vi "Strip Units__ogtk.vi"(8 "error in (no error)":errorcluster, 10 "Number or 1D array with units":variant) -> (0 "error out":errorcluster, 2 "Pure Number(s) (base units)":variant)   [LabVIEW 2023, in "openg_variant.lvlib"]
doc: "Converts a number with or without units to pure number."
uses:
  openg_variant.lvlib
  error/error.llb/openg_error.lvlib
panel:
  # "[OpenG VI Tags] ***Do Not Remove***"
  # "Please visit http://www.OpenG.org to learn about the\nOpen Source LabVIEW software movement.\n\nNOTICE -- YOU MUST LEAVE THIS NOTICE IN PLACE.  PER THE TERMS OF THE LICENSE BELOW, YOU MAY SUBLICENSE THIS SOFTWARE \nIN ANY WAY THAT DOES NOT CONFLICT WITH THIS LICENSE.\n\n### BSD License (http://www.opensource.org/licenses/bsd-license.php) Begin ###\n \nCopyright (c) 2003, Jean-Pierre Drolet <drolet_jp@hotmail.com>\nCopyright (c) 2003-2006, Jim Kring <jim@jimkring.com>\n\nAll rights reserved.\n\nRedistribution and use in source and binary forms, with or without modification, are permitted provided that the following conditions are met:\n\n    * Redistributions of source code must retain the above copyright notice, this list of conditions and the following disclaimer.\n    * Redistributions in binary form must reproduce the above copyright notice, this list of conditions and the following disclaimer in the \n       documentation and/or other materials provided with the distribution.\n    * Neither the name of SciWare, James Kring, Inc., nor the names of its contributors may be used to endorse or promote products derived \n       from this software without specific prior written permission.\n\nTHIS SOFTWARE IS PROVIDED BY THE COPYRIGHT HOLDERS AND CONTRIBUTORS \"AS IS\" AND ANY EXPRESS OR IMPLIED WARRANTIES, \nINCLUDING, BUT NOT LIMITED TO, THE IMPLIED WARRANTIES OF MERCHANTABILITY AND FITNESS FOR A PARTICULAR PURPOSE ARE \nDISCLAIMED. IN NO EVENT SHALL THE COPYRIGHT OWNER OR CONTRIBUTORS BE LIABLE FOR ANY DIRECT, INDIRECT, INCIDENTAL,\n SPECIAL, EXEMPLARY, OR CONSEQUENTIAL DAMAGES (INCLUDING, BUT NOT LIMITED TO, PROCUREMENT OF SUBSTITUTE GOODS OR \nSERVICES; LOSS OF USE, DATA, OR PROFITS; OR BUSINESS INTERRUPTION) HOWEVER CAUSED AND ON ANY THEORY OF LIABILITY, \nWHETHER IN CONTRACT, STRICT LIABILITY, OR TORT (INCLUDING NEGLIGENCE OR OTHERWISE) ARISING IN ANY WAY OUT OF THE USE \nOF THIS SOFTWARE, EVEN IF ADVISED OF THE POSSIBILITY OF SUCH DAMAGE.\n\n### BSD License End ###"
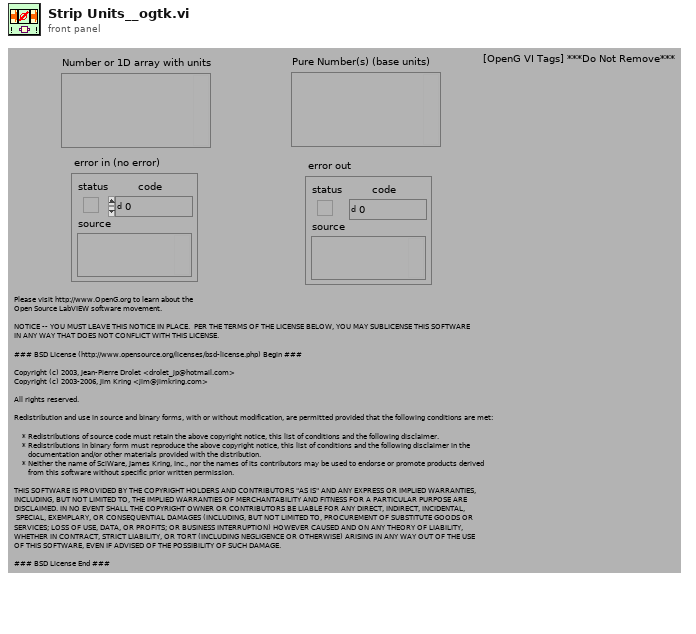
[diagram p1: front panel]
types:
  T1 = typedef "openg_variant.lvlib/Type Descriptor Header__ogtk.ctl" = cluster{"length":u16, "private":u8, "type":T2, "# elements":u16}
  T2 = typedef "openg_variant.lvlib/Type Descriptor Enumeration__ogtk.ctl" = enum8{"<Null>", "I8", "I16", "I32", "I64", "U8", "U16", "U32", "U64", "SGL", "DBL", "EXT", "CSG", "CDB", "CXT", "0x0F", "0x10", "0x11", "0x12", "0x13", "0x14", "Enum U8", "Enum U16", "Enum U32", "Enum U64", "SGL PQ", "DBL PQ", "EXT PQ", "CSG PQ", "CDB PQ", "CXT PQ", "0x1F", "0x20", "Boolean", "0x22", "0x23", "0x24", "0x25", "0x26", "0x27", "0x28", "0x29", "0x2A", "0x2B", "0x2C", "0x2D", "0x2E", "0x2F", "String", "0x31", "Path", "Pict", "0x34", "0x35", "0x36", "DAQ", "0x38", "0x39", "0x3A", "0x3B", "0x3C", "0x3D", "0x3E", "0x3F", "Array", "0x41", "0x42", "0x43", "0x44", "0x45", "0x46", "0x47", "0x48", "0x49", "0x4A", "0x4B", "0x4C", "0x4D", "0x4E", "0x4F", "Cluster", "0x51", "0x52", "Variant", "Waveform", "0x55", "0x56", "0x57", "0x58", "0x59", "0x5A", "0x5B", "0x5C", "0x5D", "0x5E", "Fixed Point", "0x60", "0x61", "0x62", "0x63", "0x64", "0x65", "0x66", "0x67", "0x68", "0x69", "0x6A", "0x6B", "0x6C", "0x6D", "0x6E", "0x6F", "Refnum", "0x71", "0x72", "Set Collection", "Map Collection"}
  T3 = typedef "openg_variant.lvlib/Type Descriptor__ogtk.ctl" = i16[]
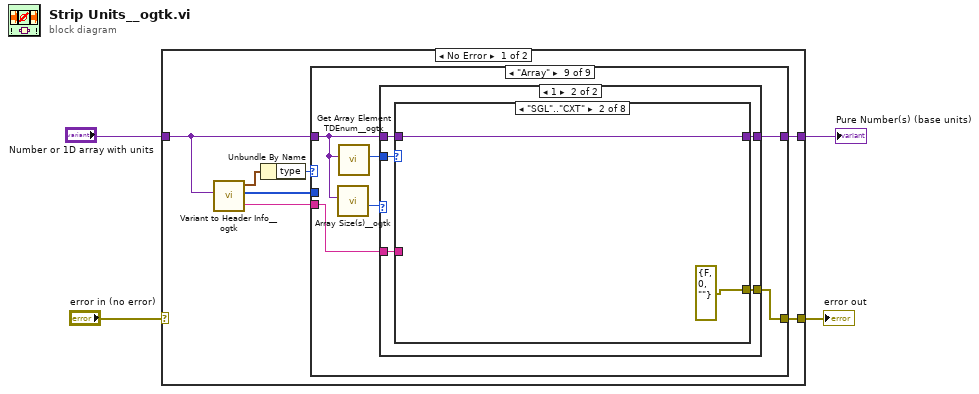
[diagram p0: block diagram]
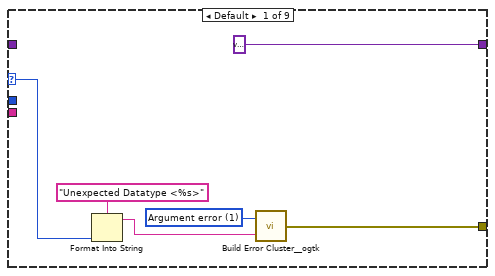
[diagram p2: hidden frame]
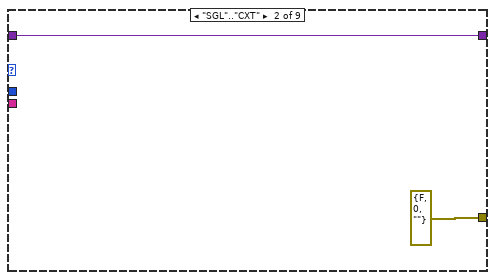
[diagram p3: hidden frame]
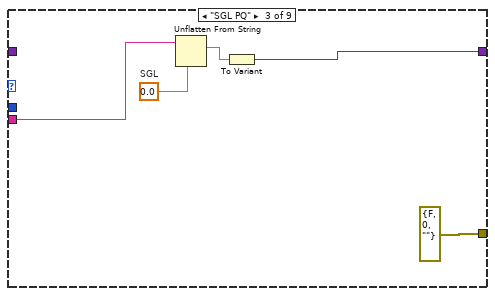
[diagram p4: hidden frame]
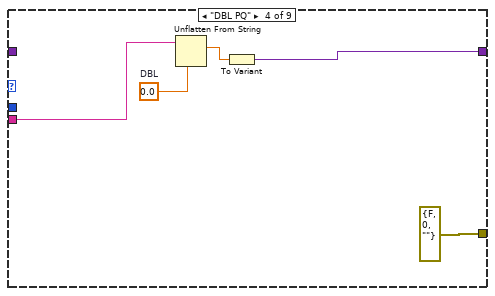
[diagram p5: hidden frame]
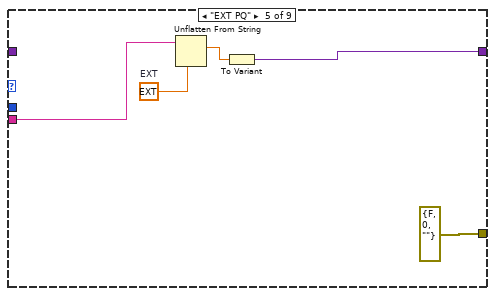
[diagram p6: hidden frame]
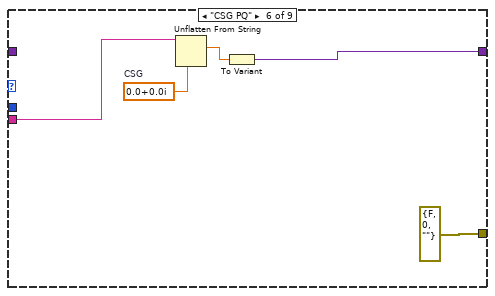
[diagram p7: hidden frame]
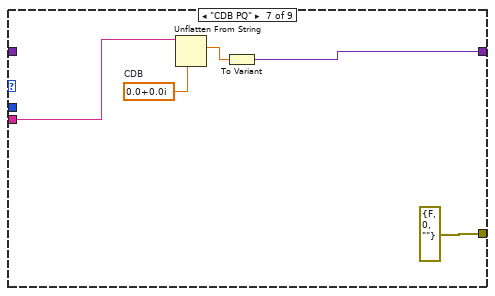
[diagram p8: hidden frame]
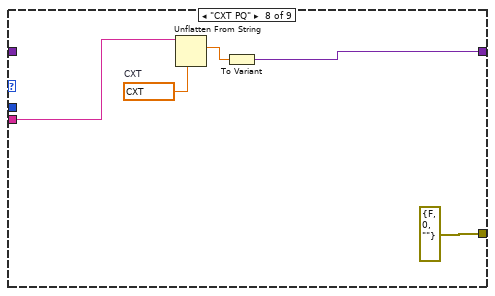
[diagram p9: hidden frame]
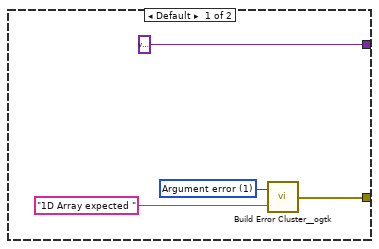
[diagram p10: hidden frame]
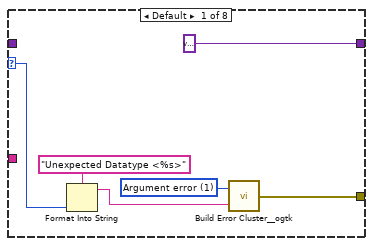
[diagram p11: hidden frame]
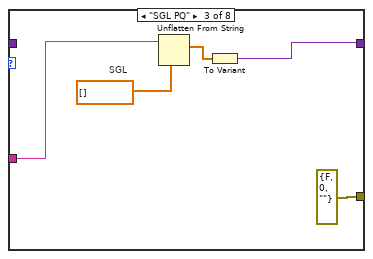
[diagram p12: hidden frame]
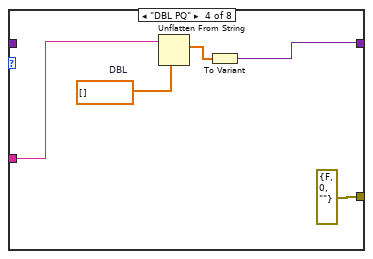
[diagram p13: hidden frame]
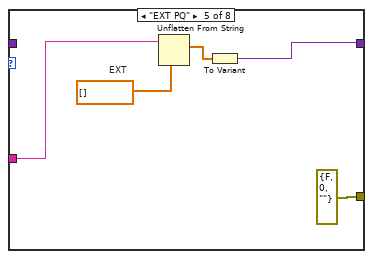
[diagram p14: hidden frame]
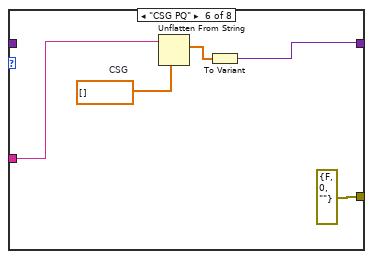
[diagram p15: hidden frame]
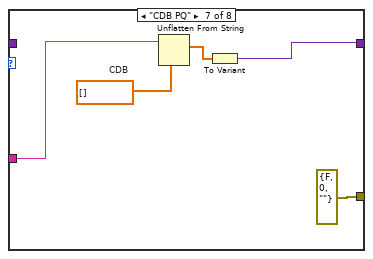
[diagram p16: hidden frame]
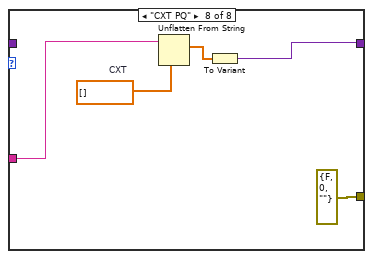
[diagram p17: hidden frame]
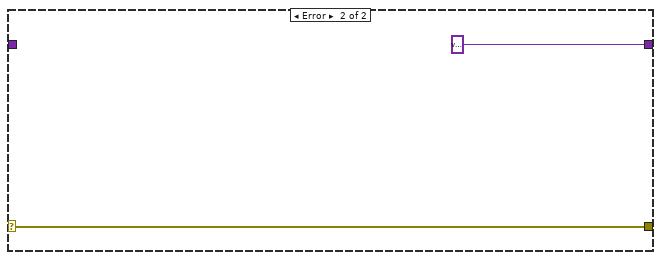
[diagram p18: hidden frame]
diagram:
  n1 = case shown="No Error" "error in (no error)" {
    selector: "error in (no error)" -> [_ w104]
    tunnel: [w11 w104] -> w4
    tunnel: "Number or 1D array with units" -> [w5 _]
    tunnel: [w6 variant ("Variant")] -> w1
    frame No Error {
      n2 = call "Variant to Header Info__ogtk.vi"("Variant"=w5) -> ("Type Descriptor Header"=w10:T1, "Type Descriptor"=w8:T3, "data string"=w7:string)  [unwired: 3 in]
      n3 = Unbundle By Name(w10) -> ("type"=w9:T2)
      n4 = case shown="\"Array\"" w9 {
        selector: w9 -> [w14 _ _ _ _ _ _ _ _]
        tunnel: [w17 errorcluster {"status"=FALSE, "code"=0, "source"=""} ("error out") errorcluster {"status"=FALSE, "code"=0, "source"=""} ("error out") errorcluster {"status"=FALSE, "code"=0, "source"=""} ("error out") errorcluster {"status"=FALSE, "code"=0, "source"=""} ("error out") errorcluster {"status"=FALSE, "code"=0, "source"=""} ("error out") errorcluster {"status"=FALSE, "code"=0, "source"=""} ("error out") errorcluster {"status"=FALSE, "code"=0, "source"=""} ("error out") w54] -> w11
        tunnel: w8 -> [_ _ _ _ _ _ _ _ _]
        tunnel: w7 -> [_ _ w20 w25 w30 w35 w40 w45 w52]
        tunnel: [variant w18 w22 w27 w32 w37 w42 w47 w53] -> w6
        tunnel: w5 -> [_ w18 _ _ _ _ _ _ w51]
        frame Default {
          w16 = 1 items=["No error", "Argument error", "Memory is full", "Out of zone", "End of file", "File already open", "Generic file I/O error", "File not found", "File permission error", "Disk is full", "Duplicate path", "Too many files open", "System feature not enabled", "Resource file not found", "Cannot add resource", "Resource not found", "Image not found", "Image memory error", "Pen does not exist", "Config type invalid", "Config token not found", "Config parse error", "Config memory error", "Bad external code format", "Bad external code offset", "External code not present", "Null window", "Destroy window error", "Null menu", "Print aborted", "Bad print record", "Print driver error", "Windows error during printing", "Memory error during printing", "Print dialog error", "Generic print error", "Invalid device refnum", "Device not found", "Device parameter error", "Device unit error", "Cannot open device", "Device call aborted", "Generic error", "Cancelled by user", "Object ID too low", "Object ID too high", "Object not in heap", "Unknown heap", "Unknown object (invalid DefProc)", "Unknown object (DefProc not in table)", "Message out of range", "Invalid (null) method", "Unknown message", "Manager call not supported", "Bad address", "Network operation in progress", "Network operation timed out", "Connection is busy", "Network attribute not supported", "Network error", "Address in use", "System out of memory", "Connection aborted", "Connection refused", "Not connected", "Already connected", "Connection closed", "Initialization error (interapplication manager)", "Bad occurrence", "Wait on unbound occurrence handler", "Occurrence queue overflow", "Datalog type conflict", "Unused", "Unrecognized type (interapplication manager)", "Memory corrupt", "Failed to make temporary DLL", "Old CIN version", "Drag socket not found", "Failed to load drop-object", "Failed to register OLE object", "Failed to release OLE object", "Format specifier type mismatch", "Unknown format specifier", "Too few format specifiers", "Too many format specifiers", "Scan failed", "Newer CIN version", "Error converting to variant", "Runtime menu error", "Password tampered", "Variant attribute not found", "Incompatible variant data type", "Event data is not available", "Event Store is not present", "Occurrence is not found", "Event Queue is not created", "Event info is not available", "Refnum passed is NULL", "Error retrieving Class GUID", "Error retrieving CoClass GUID", "Error retrieving TypeLib GUID.", "Bad built application magic bytes.", "Specific driver is different from the specific driver associated with the Logical Name.", "There is no session opened to the class driver.", "Max Error", "MAX - Error with config objects", "MAX - Error loading configuration", "MAX - Group not supported"]
          n5 = Format Into String(format string="Unexpected Datatype <%s>" ("Format String"), w14) -> (resulting string=w13:string)  [unwired: 2 in, 1 out]
          n6 = call "Build Error Cluster__ogtk.vi"("String to Prepend to source (\"\")"=w13, "code"=w16) -> ("error out"=w17:errorcluster)
        }
        frame "SGL".."CXT" {
        }
        frame "SGL PQ" {
          w24 = sgl 0.0  # SGL
          n7 = Unflatten From String(type=w24, binary string=w20) -> (value=w23:sgl)  [unwired: 3 in, 2 out]
          n8 = To Variant(anything=w23) -> (Variant=w22:variant)
        }
        frame "DBL PQ" {
          w29 = 0.0  # DBL
          n9 = Unflatten From String(type=w29, binary string=w25) -> (value=w28:dbl)  [unwired: 3 in, 2 out]
          n10 = To Variant(anything=w28) -> (Variant=w27:variant)
        }
        frame "EXT PQ" {
          w34 = ext 0.0  # EXT
          n11 = Unflatten From String(type=w34, binary string=w30) -> (value=w33:ext)  [unwired: 3 in, 2 out]
          n12 = To Variant(anything=w33) -> (Variant=w32:variant)
        }
        frame "CSG PQ" {
          w39 = csg 0.0+0.0i  # CSG
          n13 = Unflatten From String(type=w39, binary string=w35) -> (value=w38:csg)  [unwired: 3 in, 2 out]
          n14 = To Variant(anything=w38) -> (Variant=w37:variant)
        }
        frame "CDB PQ" {
          w44 = cdb 0.0+0.0i  # CDB
          n15 = Unflatten From String(type=w44, binary string=w40) -> (value=w43:cdb)  [unwired: 3 in, 2 out]
          n16 = To Variant(anything=w43) -> (Variant=w42:variant)
        }
        frame "CXT PQ" {
          w49 = cxt 0.0+0.0i  # CXT
          n17 = Unflatten From String(type=w49, binary string=w45) -> (value=w48:cxt)  [unwired: 3 in, 2 out]
          n18 = To Variant(anything=w48) -> (Variant=w47:variant)
        }
        frame "Array" {
          n19 = call "Array Size(s)__ogtk.vi"("Array"=w51) -> ("N dims"=w50:u32)  [unwired: 8 in, 2 out]
          n20 = call "Get Array Element TDEnum__ogtk.vi"("Array"=w51) -> ("Element Type"=w55:T2)  [unwired: 9 in, 1 out]
          n21 = case shown="1" w50 {
            tunnel: w55 -> [_ w64]
            tunnel: [w57 w63] -> w54
            tunnel: [variant w62] -> w53
            tunnel: w52 -> [_ w61]
            tunnel: w51 -> [_ w60]
            frame Default {
              w58 = 1 items=["No error", "Argument error", "Memory is full", "Out of zone", "End of file", "File already open", "Generic file I/O error", "File not found", "File permission error", "Disk is full", "Duplicate path", "Too many files open", "System feature not enabled", "Resource file not found", "Cannot add resource", "Resource not found", "Image not found", "Image memory error", "Pen does not exist", "Config type invalid", "Config token not found", "Config parse error", "Config memory error", "Bad external code format", "Bad external code offset", "External code not present", "Null window", "Destroy window error", "Null menu", "Print aborted", "Bad print record", "Print driver error", "Windows error during printing", "Memory error during printing", "Print dialog error", "Generic print error", "Invalid device refnum", "Device not found", "Device parameter error", "Device unit error", "Cannot open device", "Device call aborted", "Generic error", "Cancelled by user", "Object ID too low", "Object ID too high", "Object not in heap", "Unknown heap", "Unknown object (invalid DefProc)", "Unknown object (DefProc not in table)", "Message out of range", "Invalid (null) method", "Unknown message", "Manager call not supported", "Bad address", "Network operation in progress", "Network operation timed out", "Connection is busy", "Network attribute not supported", "Network error", "Address in use", "System out of memory", "Connection aborted", "Connection refused", "Not connected", "Already connected", "Connection closed", "Initialization error (interapplication manager)", "Bad occurrence", "Wait on unbound occurrence handler", "Occurrence queue overflow", "Datalog type conflict", "Unused", "Unrecognized type (interapplication manager)", "Memory corrupt", "Failed to make temporary DLL", "Old CIN version", "Drag socket not found", "Failed to load drop-object", "Failed to register OLE object", "Failed to release OLE object", "Format specifier type mismatch", "Unknown format specifier", "Too few format specifiers", "Too many format specifiers", "Scan failed", "Newer CIN version", "Error converting to variant", "Runtime menu error", "Password tampered", "Variant attribute not found", "Incompatible variant data type", "Event data is not available", "Event Store is not present", "Occurrence is not found", "Event Queue is not created", "Event info is not available", "Refnum passed is NULL", "Error retrieving Class GUID", "Error retrieving CoClass GUID", "Error retrieving TypeLib GUID.", "Bad built application magic bytes.", "Specific driver is different from the specific driver associated with the Logical Name.", "There is no session opened to the class driver.", "Max Error", "MAX - Error with config objects", "MAX - Error loading configuration", "MAX - Group not supported"]
              n22 = call "Build Error Cluster__ogtk.vi"("String to Prepend to source (\"\")"="1D Array expected " ("Format String"), "code"=w58) -> ("error out"=w57:errorcluster)
            }
            frame 1 {
              n23 = case shown="\"SGL\"..\"CXT\"" w64 {
                selector: w64 -> [w67 _ _ _ _ _ _ _]
                tunnel: [w66 errorcluster {"status"=FALSE, "code"=0, "source"=""} ("error out") errorcluster {"status"=FALSE, "code"=0, "source"=""} ("error out") errorcluster {"status"=FALSE, "code"=0, "source"=""} ("error out") errorcluster {"status"=FALSE, "code"=0, "source"=""} ("error out") errorcluster {"status"=FALSE, "code"=0, "source"=""} ("error out") errorcluster {"status"=FALSE, "code"=0, "source"=""} ("error out") errorcluster {"status"=FALSE, "code"=0, "source"=""} ("error out")] -> w63
                tunnel: [variant ("Variant") w72 w74 w79 w84 w89 w94 w99] -> w62
                tunnel: w60 -> [_ w72 _ _ _ _ _ _]
                tunnel: w61 -> [_ _ w75 w80 w85 w90 w95 w100]
                frame Default {
                  w70 = 1 items=["No error", "Argument error", "Memory is full", "Out of zone", "End of file", "File already open", "Generic file I/O error", "File not found", "File permission error", "Disk is full", "Duplicate path", "Too many files open", "System feature not enabled", "Resource file not found", "Cannot add resource", "Resource not found", "Image not found", "Image memory error", "Pen does not exist", "Config type invalid", "Config token not found", "Config parse error", "Config memory error", "Bad external code format", "Bad external code offset", "External code not present", "Null window", "Destroy window error", "Null menu", "Print aborted", "Bad print record", "Print driver error", "Windows error during printing", "Memory error during printing", "Print dialog error", "Generic print error", "Invalid device refnum", "Device not found", "Device parameter error", "Device unit error", "Cannot open device", "Device call aborted", "Generic error", "Cancelled by user", "Object ID too low", "Object ID too high", "Object not in heap", "Unknown heap", "Unknown object (invalid DefProc)", "Unknown object (DefProc not in table)", "Message out of range", "Invalid (null) method", "Unknown message", "Manager call not supported", "Bad address", "Network operation in progress", "Network operation timed out", "Connection is busy", "Network attribute not supported", "Network error", "Address in use", "System out of memory", "Connection aborted", "Connection refused", "Not connected", "Already connected", "Connection closed", "Initialization error (interapplication manager)", "Bad occurrence", "Wait on unbound occurrence handler", "Occurrence queue overflow", "Datalog type conflict", "Unused", "Unrecognized type (interapplication manager)", "Memory corrupt", "Failed to make temporary DLL", "Old CIN version", "Drag socket not found", "Failed to load drop-object", "Failed to register OLE object", "Failed to release OLE object", "Format specifier type mismatch", "Unknown format specifier", "Too few format specifiers", "Too many format specifiers", "Scan failed", "Newer CIN version", "Error converting to variant", "Runtime menu error", "Password tampered", "Variant attribute not found", "Incompatible variant data type", "Event data is not available", "Event Store is not present", "Occurrence is not found", "Event Queue is not created", "Event info is not available", "Refnum passed is NULL", "Error retrieving Class GUID", "Error retrieving CoClass GUID", "Error retrieving TypeLib GUID.", "Bad built application magic bytes.", "Specific driver is different from the specific driver associated with the Logical Name.", "There is no session opened to the class driver.", "Max Error", "MAX - Error with config objects", "MAX - Error loading configuration", "MAX - Group not supported"]
                  n24 = Format Into String(format string="Unexpected Datatype <%s>" ("Format String"), w67) -> (resulting string=w68:string)  [unwired: 2 in, 1 out]
                  n25 = call "Build Error Cluster__ogtk.vi"("String to Prepend to source (\"\")"=w68, "code"=w70) -> ("error out"=w66:errorcluster)
                }
                frame "SGL".."CXT" {
                }
                frame "SGL PQ" {
                  w76 = sgl[] []  # SGL
                  n26 = Unflatten From String(type=w76, binary string=w75) -> (value=w77:sgl[])  [unwired: 3 in, 2 out]
                  n27 = To Variant(anything=w77) -> (Variant=w74:variant)
                }
                frame "DBL PQ" {
                  w81 = dbl[] []  # DBL
                  n28 = Unflatten From String(type=w81, binary string=w80) -> (value=w82:dbl[])  [unwired: 3 in, 2 out]
                  n29 = To Variant(anything=w82) -> (Variant=w79:variant)
                }
                frame "EXT PQ" {
                  w86 = ext[] []  # EXT
                  n30 = Unflatten From String(type=w86, binary string=w85) -> (value=w87:ext[])  [unwired: 3 in, 2 out]
                  n31 = To Variant(anything=w87) -> (Variant=w84:variant)
                }
                frame "CSG PQ" {
                  w91 = csg[] []  # CSG
                  n32 = Unflatten From String(type=w91, binary string=w90) -> (value=w92:csg[])  [unwired: 3 in, 2 out]
                  n33 = To Variant(anything=w92) -> (Variant=w89:variant)
                }
                frame "CDB PQ" {
                  w96 = cdb[] []  # CDB
                  n34 = Unflatten From String(type=w96, binary string=w95) -> (value=w97:cdb[])  [unwired: 3 in, 2 out]
                  n35 = To Variant(anything=w97) -> (Variant=w94:variant)
                }
                frame "CXT PQ" {
                  w101 = cxt[] []  # CXT
                  n36 = Unflatten From String(type=w101, binary string=w100) -> (value=w102:cxt[])  [unwired: 3 in, 2 out]
                  n37 = To Variant(anything=w102) -> (Variant=w99:variant)
                }
              }
            }
          }
        }
      }
    }
    frame Error {
    }
  }
  "error out" <- w4
  "Pure Number(s) (base units)" <- w1
